vi "RunOperation.vi"(10 "Inputs":string[](array[string])=["", ""], 11 "AddNum in":refnum<class "AddTwoNumbers.lvclass">) -> (1 "Output/Failure":string, 2 "CLI Process Return Code":i32, 3 "AddNum out":refnum<class "AddTwoNumbers.lvclass">)   [LabVIEW 2014, in "AddTwoNumbers.lvclass"]
doc: "This operation vi adds two number for valid inputs."
uses:
  AddTwoNumbers.lvclass
  Program Files (x86)/National Instruments/Shared/LabVIEW CLI/Operations/Utilities/Logger/Logger.lvclass
panel:
  # "Overview: This VI demonstrates how to define the behavior of the AddNum operation.\n\nInstructions:\n1. Open the block diagram.\n2. Review the code and the block diagram comments. Try to understand how each section of code affects the behavior of this operation.\n3. (Optional) Run this operation in the command line interface (CLI) for LabVIEW. Check if the operation works as expected.\n     For example, you can run this operation by executing the LabVIEW CLI -OperationName AddTwoNumbers 23 45 command. Check if the CLI for LabVIEW returns 68.\n4. Open command prompt and run AddTwoNumbers.bat. Or, examine RunVIExampleScript.bat. \n\nFor more information about creating a custom operation, refer to the Creating Custom Command Line Operations topic in the LabVIEW Help, available from Help>>LabVIEW Help."
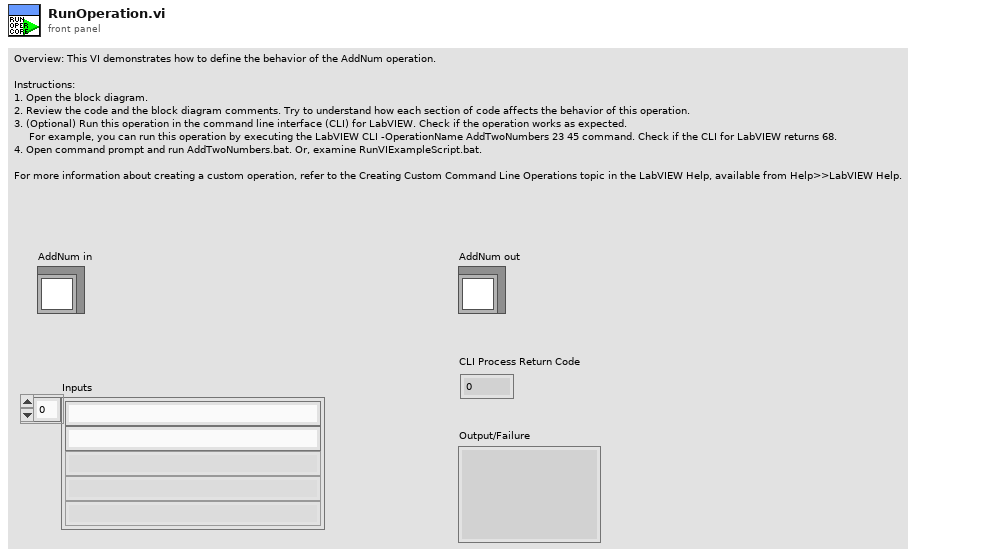
[diagram p1: front panel]
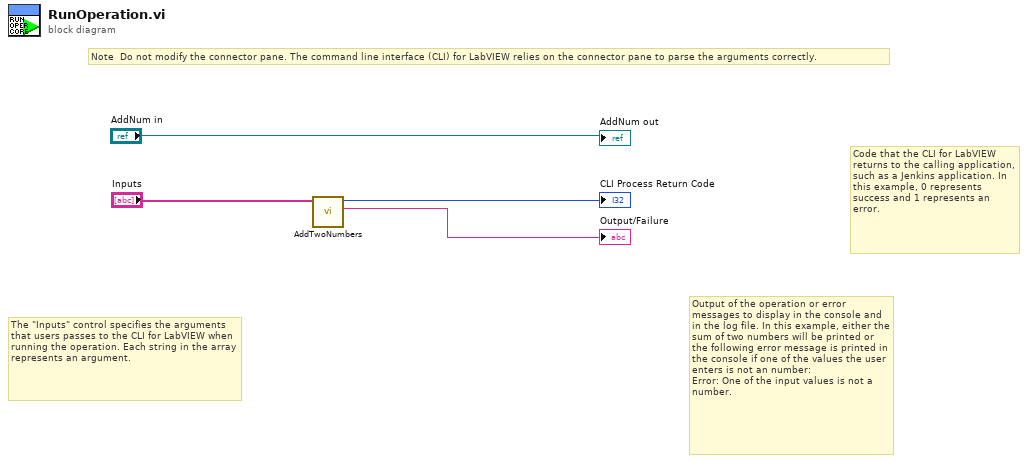
[diagram p0: block diagram]
diagram:
  # "Output of the operation or error messages to display in the console and in the log file. In this example, either the sum of two numbers will be printed or the following error message is printed in the console if one of the values the user enters is not an number:\nError: One of the input values is not a number."
  # "Code that the CLI for LabVIEW returns to the calling application, such as a Jenkins application. In this example, 0 represents success and 1 represents an error."
  # "The \"Inputs\" control specifies the arguments that users passes to the CLI for LabVIEW when running the operation. Each string in the array represents an argument."
  # "Note  Do not modify the connector pane. The command line interface (CLI) for LabVIEW relies on the connector pane to parse the arguments correctly."
  n1 = call "AddTwoNumbers.vi"("Inputs"="Inputs") -> ("Output/Failure"=→"Output/Failure":string, "CLI Process Return Code"=→"CLI Process Return Code":i32)  [unwired: 9 in]
  "AddNum out" <- "AddNum in"
